vi "Read Valve Pos.vi"(8 "error in (no error)":errorcluster) -> (0 "error out":errorcluster)   [LabVIEW 2018, in "PHD Ultra.lvlib" / "PHD Ultra.lvclass"]
uses:
  PHD Ultra.lvclass
  Resources/GLOBAL/GLOBAL Time-critical.vi
  <userlib>/QmixLib/QmixLib.lvlib
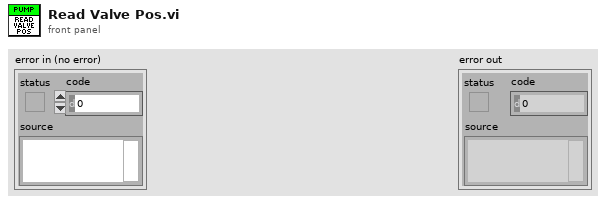
[diagram p1: front panel]
types:
  T1 = enum16{"LOW_PRESSURE_VALVE", "BALL_VALVE", "QMIX_VALVE"}
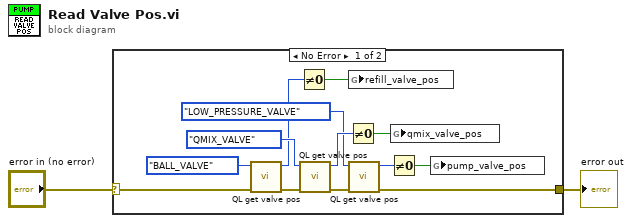
[diagram p0: block diagram]
diagram:
  n1 = case shown="No Error" "error in (no error)" {
    selector: "error in (no error)" -> [w6 w16]
    tunnel: [w3 w16] -> w1
    frame No Error {
      n2 = call <userlib>:"QL get valve pos.vi"("error in (no error) 2"=w6, "valve"=T1."BALL_VALVE") -> ("error out 2"=w5:errorcluster, "pos"=w8:i32)  [unwired: 8 in]
      n3 = Not Equal To 0?(x=w8) -> (x != 0?=w7:bool)
      n4 = call <userlib>:"QL get valve pos.vi"("error in (no error) 2"=w5, "valve"=T1."QMIX_VALVE") -> ("error out 2"=w4:errorcluster, "pos"=w13:i32)  [unwired: 8 in]
      n5 = Not Equal To 0?(x=w13) -> (x != 0?=w12:bool)
      n6 = global write "GLOBAL Time-critical.vi" "refill_valve_pos"(w7) -> ()
      n7 = call <userlib>:"QL get valve pos.vi"("error in (no error) 2"=w4, "valve"=T1."LOW_PRESSURE_VALVE") -> ("error out 2"=w3:errorcluster, "pos"=w10:i32)  [unwired: 8 in]
      n8 = Not Equal To 0?(x=w10) -> (x != 0?=w9:bool)
      n9 = global write "GLOBAL Time-critical.vi" "qmix_valve_pos"(w12) -> ()
      n10 = global write "GLOBAL Time-critical.vi" "pump_valve_pos"(w9) -> ()
    }
    frame Error {
    }
  }
  "error out" <- w1
